vi "Configuration Read.vi"(8 "error in (no error)":errorcluster, 11 "NI DMM Driver in":refnum<class "DMM.NI.lvclass">) -> (0 "error out":errorcluster, 1 "Range":dbl, 2 "Function":T2, 3 "NI DMM Driver out":refnum<class "DMM.NI.lvclass">, 5 "Digit Resolution(5½)":T1=enum."5½")   [LabVIEW 2020, in "NI DMM Driver.lvlib" / "DMM.NI.lvclass"]
doc: "Read the DMM configuration: Function, Range and Resolution."
uses:
  DMM.NI.lvclass
  PPL/HDH.Driver.DMM.lvlibp/Controls/Ctl_Function.ctl
  PPL/HDH.Driver.DMM.lvlibp/Controls/Ctl_DigitResolution.ctl
  DMM.NI.lvclass/DMM.NI.ctl
  PPL/HDH.Driver.DMM.lvlibp
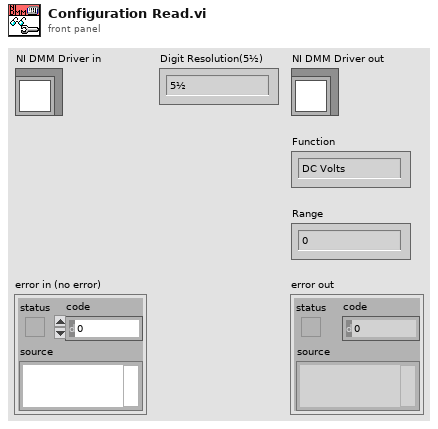
[diagram p1: front panel]
types:
  T1 = typedef "HDH.Driver.DMM.lvlibp/Ctl_DigitResolution.ctl" = enum8{"3½", "4½", "5½", "6½", "7½"}
  T2 = typedef "HDH.Driver.DMM.lvlibp/Ctl_Function.ctl" = enum8{"DC Volts", "AC Volts", "DC Current", "AC Current", "2-wire Resistance", "4-wire Resistance", "Diode", "Frequency", "Period", "AC Volts DC Coupled", "Capacitance", "Inductance", "Temperature"}
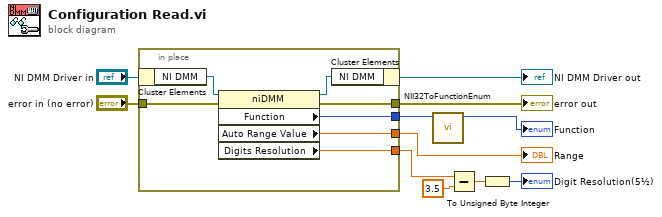
[diagram p0: block diagram]
diagram:
  n1 = in-place {
    in-place-border: "error in (no error)" -> [w16]
    in-place-border: [w15] -> w8
    in-place-border: [w14] -> w6
    in-place-border: [w13] -> w5
    in-place-border: [w12] -> w1
    n2 = in-place-cluster #1("NI DMM Driver in") -> ("NI DMM"=w18:refnum<k15>)
    n3 = property class="niDMM"(reference=w18, error in=w16) -> (reference out=w17:refnum<k15>, error out=w12:errorcluster, "Function"=w15:i32, "Auto Range Value"=w14:dbl, "Digits Resolution"=w13:dbl)
    n4 = in-place-cluster #1("NI DMM"=w17) -> (→"NI DMM Driver out":refnum<class "DMM.NI.lvclass">)
  }
  "error out" <- w1
  "Range" <- w6
  n5 = call "NII32ToFunctionEnum.vi"("NI Function in"=w8) -> ("Function out"=→"Function":T2)  [unwired: 10 in]
  n6 = Subtract(x=w5, y=3.5) -> (x-y=w3:dbl)
  n7 = To Unsigned Byte Integer(number=w3) -> (unsigned 8bit integer=→"Digit Resolution(5½)":u8)
